vi "SetCurrentPollCommandStatusToCVT.vi"(7 "Complete":bool, 8 "error in (no error)":errorcluster, 9 "Ack":i32, 10 "Command":string, 11 "Data Value Reference in":T1) -> (0 "error out":errorcluster, 3 "Data Value Reference out":T1)   [LabVIEW 2022 SP3, in "GIS Printer.lvclass"]
uses:
  GIS Printer.lvclass
  <vilib>/TELLC/Dynamic CVT API/TD Dynamic CVT DVR--ref.ctl
  Typedefs/PollCommandData-Cluster.ctl
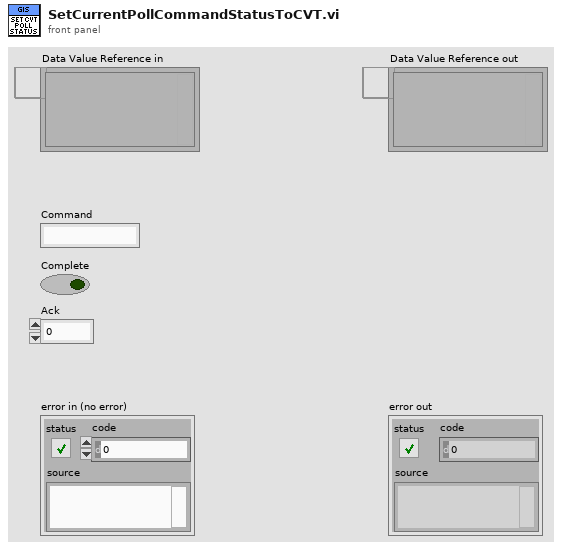
[diagram p1: front panel]
types:
  T1 = typedef "TD Dynamic CVT DVR--ref.ctl" = refnum<data-value>
  T2 = typedef "PollCommandData-Cluster.ctl" = cluster{"Command":string, "ID":i32, "Complete":bool}
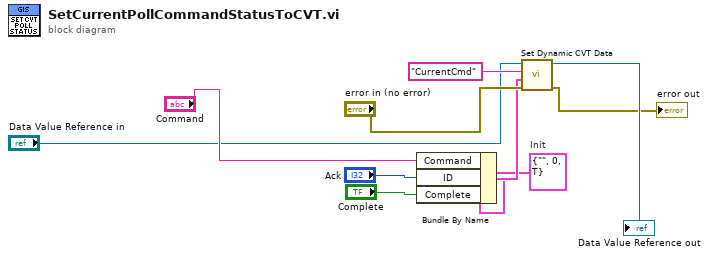
[diagram p0: block diagram]
diagram:
  w2 = T2 {"Command"="", "ID"=0, "Complete"=TRUE}  # Init
  n1 = Bundle By Name(cluster=w2, "Command"="Command", "ID"="Ack", "Complete"="Complete") -> (w5:T2)
  n2 = call <vilib>:"Set Dynamic CVT Data.vi"("error in (no error)"="error in (no error)", "value"=w5, "DataName"="CurrentCmd", "dCVT DVR"="Data Value Reference in") -> ("error out"=→"error out":errorcluster, "dCVT DVR out"=→"Data Value Reference out":T1)  [unwired: 5 in, 1 out]
